vi "ECOG-Settings Dialog.vi"(0 "Settings in":T2, 2 "Parent VI":refnum<vi>) -> (4 "Settings out":T2, 10 "canceled":bool)   [LabVIEW 2020]
uses:
  Typedefs/ECOG-Parameters.ctl
  epl-vi-lib/Utility VIs/Buttons/KCheckmarkBoolean 2.ctl
panel:
  in  "Fhi (Hz)":dbl
  in  "Flo (Hz)":dbl
  in  "Filter":T1
  in  "History Length (s)":dbl
  in  "Frame Size (ms)":dbl
  in  "Sample Rate (Hz)":dbl
  in  "Channel":u16(ring) items=["PXI1Slot4/ai0", "PXI1Slot4/ai1", "PXI1Slot4/ai2", "PXI1Slot4/ai3", "PXI1Slot4/ai4", "PXI1Slot4/ai5", "PXI1Slot4/ai6", "PXI1Slot4/ai7"]
  in  "Cancel":bool
  in  "OK":bool
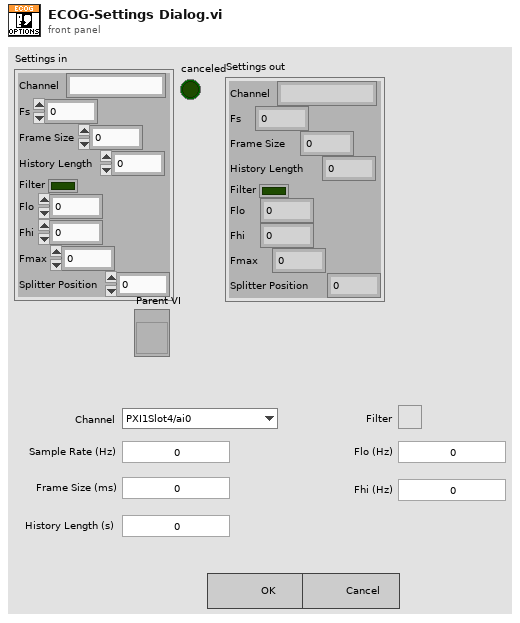
[diagram p1: front panel]
types:
  T1 = typedef "KCheckmarkBoolean 2.ctl" = bool
  T2 = typedef "ECOG-Parameters.ctl" = cluster{"Channel":string, "Fs":dbl, "Frame Size":dbl, "History Length":dbl, "Filter":bool, "Flo":dbl, "Fhi":dbl, "Fmax":dbl, "Splitter Position":i32}
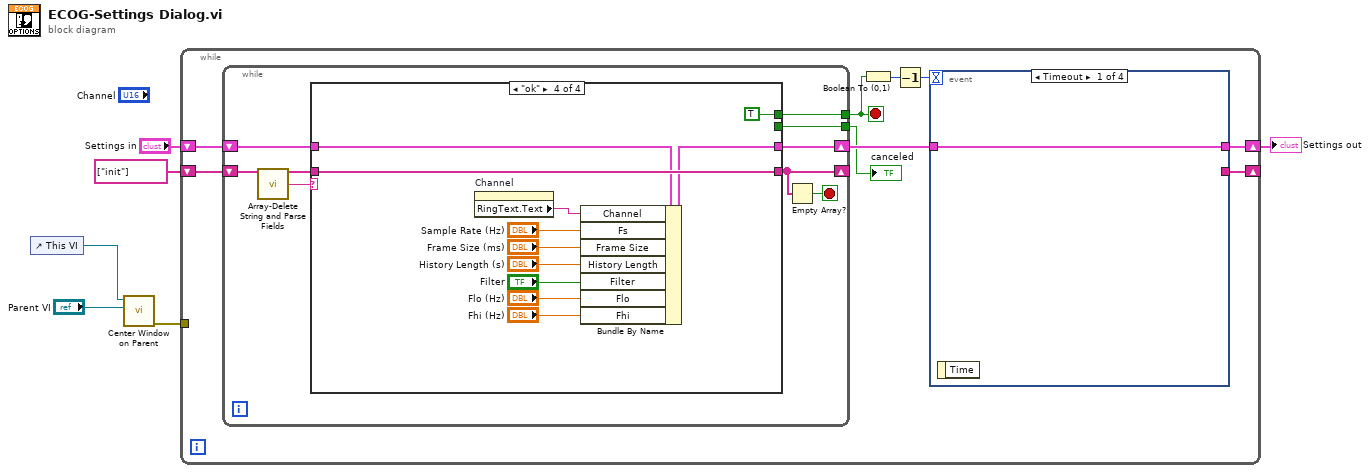
[diagram p0: block diagram]
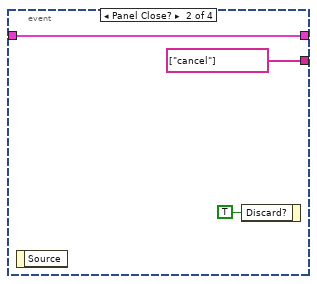
[diagram p2: hidden frame]
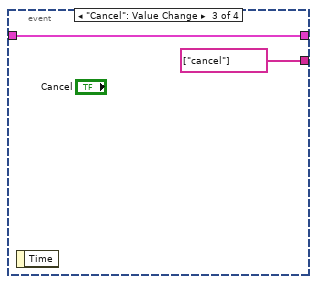
[diagram p3: hidden frame]
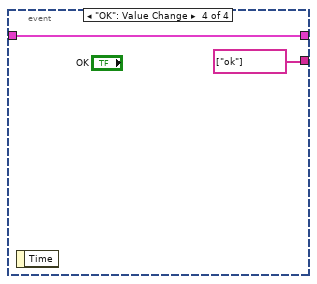
[diagram p4: hidden frame]
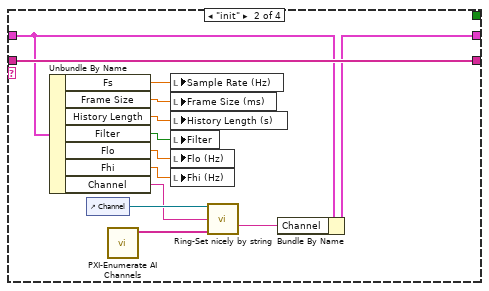
[diagram p6: hidden frame]
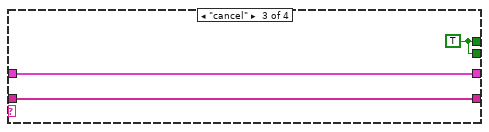
[diagram p7: hidden frame]
diagram:
  n1 = control-ref of="This VI"() -> (w1:refnum<vi>)
  n2 = call "Center Window on Parent.vi"("Parent VI"="Parent VI", "VI in"=w1) -> ("error out"=w3:errorcluster)  [unwired: 8 in, 1 out]
  n3 = while {
    shift-right: [w9] -> w5
    shift-left: "Settings in" -> [w15]
    shift-right: [w8] -> _
    shift-left: string[] ["init"] -> [w10]
    tunnel: w3 -> [_]
    stop <- w13 stop-if-true
    n4 = while {
      shift-right: [w31] -> _
      shift-left: w10 -> [w25]
      shift-right: [w28] -> w14
      shift-left: w15 -> [w29]
      tunnel: [w27] -> w13
      tunnel: [w24] -> w7
      stop <- w30 stop-if-true
      n5 = call "Array-Delete String and Parse Fields.vi"("Array in"=w25) -> ("Array out"=w32:string[], "Field 1"=w26:string)  [unwired: 10 in, 3 out]
      n6 = case shown="\"ok\"" w26 {
        tunnel: w32 -> [w34 w47 w50 w61]
        tunnel: [w34 w47 w50 w61] -> w31
        tunnel: w29 -> [w33 w46 w49 w60]
        tunnel: [w33 w40 w49 w58] -> w28
        tunnel: [_ _ w48 TRUE] -> w27
        tunnel: [_ _ w48 _] -> w24
        frame "", Default {
        }
        frame "init" {
          n7 = Unbundle By Name(w46) -> ("Fs"=w45:dbl, "Frame Size"=w44:dbl, "History Length"=w43:dbl, "Filter"=w37:bool, "Flo"=w36:dbl, "Fhi"=w35:dbl, "Channel"=w41:string)
          n8 = control-ref of="Channel"() -> (w42:refnum<vi>)
          n9 = call "PXI-Enumerate AI Channels.vi"() -> ("AI.PhysicalChans"=w38:tag[])  [unwired: 11 in]
          n10 = local write "Sample Rate (Hz)"(w45) -> ()
          n11 = local write "Frame Size (ms)"(w44) -> ()
          n12 = local write "History Length (s)"(w43) -> ()
          n13 = local write "Filter"(w37) -> ()
          n14 = local write "Flo (Hz)"(w36) -> ()
          n15 = local write "Fhi (Hz)"(w35) -> ()
          n16 = call "Ring-Set nicely by string.vi"("Ring in"=w42, "Device"=w41, "Strings []"=w38) -> ("Selection"=w39:string)  [unwired: 8 in, 4 out]
          n17 = Bundle By Name(cluster=w46, "Channel"=w39) -> (w40:T2)
        }
        frame "cancel" {
          w48 = TRUE
        }
        frame "ok" {
          n18 = property on="Channel" class="Ring (strict)"() -> ("RingText.Text"=w57:string)  [unwired: 2 in, 2 out]
          n19 = Bundle By Name(cluster=w60, "Channel"=w57, "Fs"="Sample Rate (Hz)", "Frame Size"="Frame Size (ms)", "History Length"="History Length (s)", "Filter"="Filter", "Flo"="Flo (Hz)", "Fhi"="Fhi (Hz)") -> (w58:T2)
        }
      }
      n20 = Empty Array?(array=w31) -> (empty?=w30:bool)
    }
    "canceled" <- w7
    n21 = Boolean To (0,1)(Boolean=w13) -> (0, 1=w12:i16)
    n22 = Decrement(x=w12) -> (x-1=w11:i16)
    n23 = event shown="[0] Timeout" {
      selector: _ -> [_ _ _ _]
      dyn-events: _ -> [_ _ _ _]
      timeout: w11 -> [_ _ _ _]
      tunnel: w14 -> [w16 w19 w20 w23]
      tunnel: [w16 w19 w20 w23] -> w9
      tunnel: [_ string[] ["cancel"] string[] ["cancel"] string[] ["ok"]] -> w8
      event Timeout {
        n24 = event-data() -> ()  [unwired: 1 in, 1 out]
      }
      event Panel Close? {
        n25 = event-data() -> ()  [unwired: 1 in, 1 out]
        n26 = event-data("Discard?"=TRUE) -> ()  [unwired: 1 in, 1 out]
      }
      event "Cancel": Value Change {
        n27 = event-data() -> ()  [unwired: 1 in, 1 out]
      }
      event "OK": Value Change {
        n28 = event-data() -> ()  [unwired: 1 in, 1 out]
      }
    }
  }
  "Settings out" <- w5
